vi "Read Configuration.vi"(7 "INI Fomatted Cluster Type":variant, 8 "error in (no error)":errorcluster, 11 "Configuration in":refnum<class "Configuration.lvclass">) -> (0 "error out":errorcluster, 2 "Configuration":variant, 3 "Configuration out":refnum<class "Configuration.lvclass">)   [LabVIEW 2016, in "Configuration.lvclass"]
uses:
  Configuration.lvclass
  Configuration.lvclass/Configuration.ctl
  <vilib>/Utility/config.llb/NI_LVConfig.lvlib
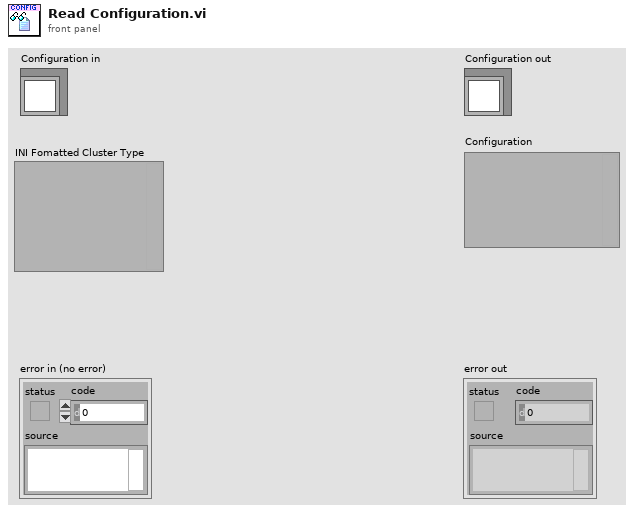
[diagram p1: front panel]
types:
  T1 = typedef "NI_LVConfig.lvlib/Config Data RefNum.ctl" = refnum<k1>
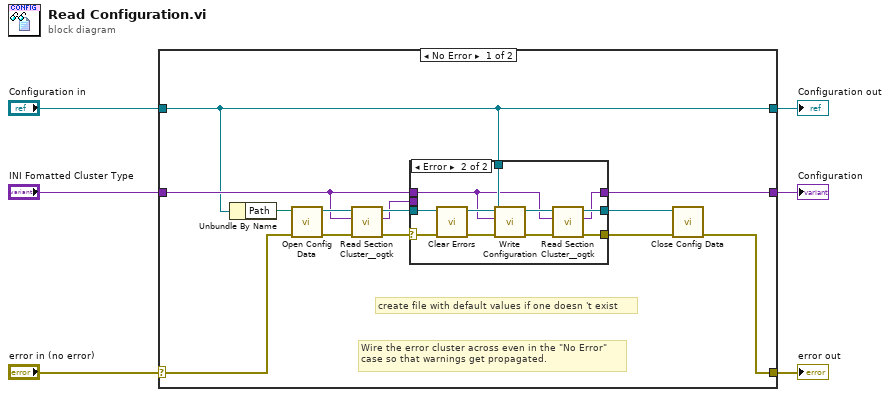
[diagram p0: block diagram]
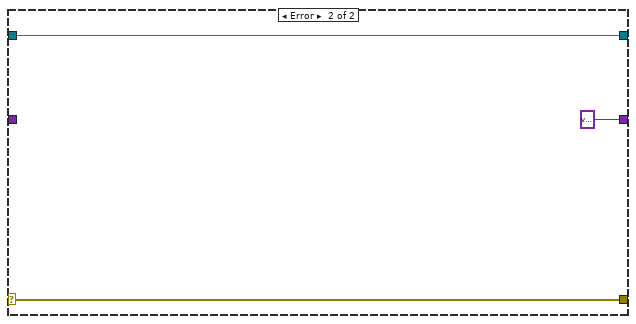
[diagram p3: hidden frame]
diagram:
  n1 = case shown="No Error" "error in (no error)" {
    selector: "error in (no error)" -> [w19 w34]
    tunnel: [w16 w34] -> w6
    tunnel: [w7 w33] -> w5
    tunnel: "Configuration in" -> [w7 w33]
    tunnel: [w10 variant ("Variant")] -> w4
    tunnel: "INI Fomatted Cluster Type" -> [w11 _]
    frame No Error {
      # "create file with default values if one doesn\t't exist"
      # "Wire the error cluster across even in the \"No Error\"\ncase so that warnings get propagated."
      n2 = Unbundle By Name(w7) -> ("Path"=w15:path)
      n3 = call <vilib>:"Open Config Data.vi"("error in (no error)"=w19, "configuration file path"=w15) -> ("error out"=w17:errorcluster, "refnum"=w18:T1)  [unwired: 7 in, 1 out]
      n4 = call <userlib>:"Read Section Cluster__ogtk.vi"("error in (no error)"=w17, "Section Formatted Cluster Type"=w11, "refnum"=w18) -> ("error out"=w8:errorcluster, "Section Formatted Cluster"=w9:variant, "dup refnum"=w14:T1)  [unwired: 4 in, 2 out]
      n5 = case shown="Error" w8 {
        selector: w8 -> [w20 w23]
        tunnel: w11 -> [_ w26]
        tunnel: w14 -> [w22 w27]
        tunnel: [w22 w30] -> w13
        tunnel: [w20 w31] -> w12
        tunnel: [w21 w29] -> w10
        tunnel: w9 -> [w21 _]
        tunnel: w7 -> [_ w28]
        frame No Error {
        }
        frame Error {
          n6 = call <vilib>:"Clear Errors.vi"("error in (no error)"=w23) -> ("error out"=w24:errorcluster)  [unwired: 5 in, 1 out]
          n7 = call "Write Configuration.vi"("error in (no error)"=w24, "Variant"=w26, "Configuration in"=w28) -> ("error out"=w25:errorcluster)  [unwired: 7 in, 1 out]
          n8 = call <userlib>:"Read Section Cluster__ogtk.vi"("error in (no error)"=w25, "Section Formatted Cluster Type"=w26, "refnum"=w27) -> ("error out"=w31:errorcluster, "Section Formatted Cluster"=w29:variant, "dup refnum"=w30:T1)  [unwired: 4 in, 2 out]
        }
      }
      n9 = call <vilib>:"Close Config Data.vi"("error in (no error)"=w12, "refnum"=w13) -> ("error out"=w16:errorcluster)  [unwired: 8 in, 1 out]
    }
    frame Error {
    }
  }
  "error out" <- w6
  "Configuration out" <- w5
  "Configuration" <- w4
